vi "RC_Client Client 2.vi"(8 "error in (no error)":errorcluster) -> (0 "error out":errorcluster)   [LabVIEW 2019, in "RemoteControl.lvlib" / "RemoteControl.lvclass"]
uses:
  RemoteControl.lvclass
  a9d26567-5b45-42ca-bcd0-d9a82bf46199.vi
panel:
  in  "RemoteControl in":refnum<class "RemoteControl.lvclass">
  in  "milliseconds to wait":u32
  out "time (1 message) (ms)":u32
  out "messsages/s":dbl
  in  "remote port":u16=6341
  in  "address":string
  out "Parse Response":string
  out "Messages":i32
  in  "Stop":bool
  out "Command reponse":string
  out "Command":string
  out "commands":string[](array[string])
  # "CLIENT (API)"
  # "Connection info"
  # "Message Sent"
  # "Message Received"
  # "Metrics"
  # "client 2"
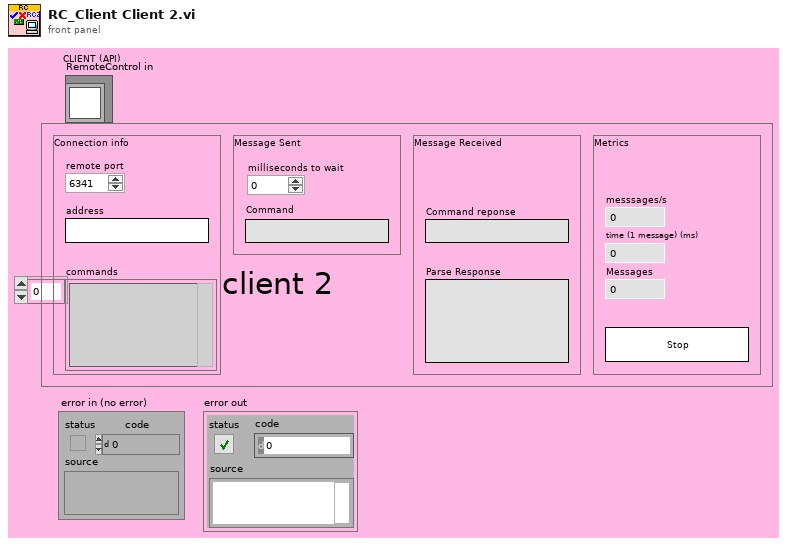
[diagram p1: front panel]
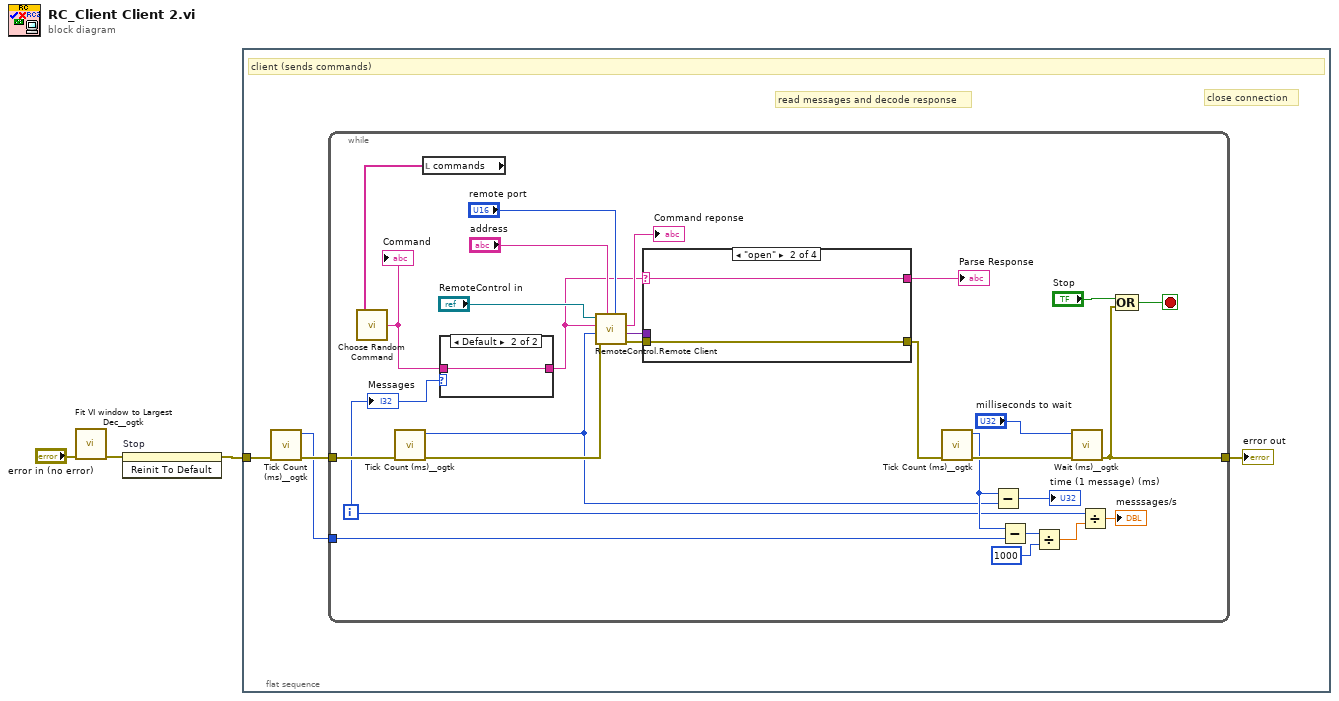
[diagram p0: block diagram]
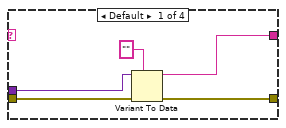
[diagram p2: hidden frame]
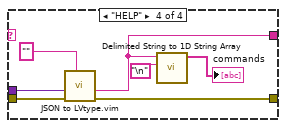
[diagram p4: hidden frame]
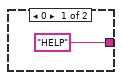
[diagram p5: hidden frame]
diagram:
  n1 = call <userlib>:"Fit VI window to Largest Dec__ogtk.vi"("error in (no error)"="error in (no error)") -> ("error out"=w3:errorcluster)  [unwired: 5 in, 1 out]
  n2 = invoke on="Stop" class="Bool" method="Reinit To Default"(error in=w3) -> (error out=w2:errorcluster)  [unwired: 2 in, 2 out]
  n3 = flat-sequence {
    tunnel: w2 -> [w4]
    frame #0 {
      # "close connection"
      # "read messages and decode response"
      # "client (sends commands)"
      n4 = call <userlib>:"Tick Count (ms)__ogtk.vi"("error in (no error)"=w4) -> ("error out"=w7:errorcluster, "millisecond timer value"=w6:u32)  [unwired: 9 in]
      n5 = while {
        tunnel: [w28] -> w5
        tunnel: w7 -> [w31]
        tunnel: w6 -> [w23]
        i -> [w20]
        stop <- w34 stop-if-true
        n6 = call <userlib>:"Tick Count (ms)__ogtk.vi"("error in (no error)"=w31) -> ("error out"=w21:errorcluster, "millisecond timer value"=w14:u32)  [unwired: 9 in]
        n7 = local read "commands"() -> (w16:string[])
        n8 = call "Choose Random Command.vi"("Array"=w16) -> ("String"=w15:string)
        "Command" <- w15
        n9 = case shown="Default" w20 {
          tunnel: ["HELP" ("Command") w52] -> w8
          tunnel: w15 -> [_ w52]
          frame 0 {
          }
          frame Default {
          }
        }
        n10 = call "RemoteControl.Remote Client.vi"("Port"="remote port", "address"="address", "error in (no error)"=w21, "Data"=w14, "Command"=w8, "RemoteControl in"="RemoteControl in") -> ("error out"=w11:errorcluster, "Data out"=w12:variant, "Command out"=→"Command reponse":string)  [unwired: 2 in, 1 out]
        n11 = case shown="\"open\"" w8 {
          selector: w8 -> [_ w40 w42 _]
          tunnel: [w35 w40 w42 w44] -> w10
          tunnel: w12 -> [w39 _ _ w48]
          tunnel: [w36 w41 w43 w45] -> w9
          tunnel: w11 -> [w37 w41 w43 w46]
          frame Default {
            n12 = Variant To Data(error in=w37, type="", Variant=w39) -> (data=w35:string, error out=w36:errorcluster)
          }
          frame "open" {
          }
          frame "close" {
          }
          frame "HELP" {
            n13 = call "JSON to LVtype.vim"("type"="", "error in (no error)"=w46, "JSON Data in"=w48) -> ("error out"=w45:errorcluster, "Data out"=w44:string)  [unwired: 7 in]
            n14 = call <vilib>:"Delimited String to 1D String Array.vi"("delimiter"="\n", "delimited string"=w44) -> ("string array"=→"commands":string[])  [unwired: 9 in]
          }
        }
        "Parse Response" <- w10
        n15 = call <userlib>:"Tick Count (ms)__ogtk.vi"("error in (no error)"=w9) -> ("error out"=w30:errorcluster, "millisecond timer value"=w25:u32)  [unwired: 9 in]
        n16 = Subtract(x=w25, y=w14) -> (x-y=→"time (1 message) (ms)":u32)
        n17 = Subtract(x=w25, y=w23) -> (x-y=w24:u32)
        n18 = Divide(x=w24, y=u32 1000) -> (x/y=w33:dbl)
        n19 = call <userlib>:"Wait (ms)__ogtk.vi"("error in (no error)"=w30, "milliseconds to wait"="milliseconds to wait") -> ("error out"=w28:errorcluster)  [unwired: 8 in, 1 out]
        n20 = Divide(x=w20, y=w33) -> (x/y=→"messsages/s":dbl)
        n21 = Compound Arithmetic op=OR("Stop", w28) -> (w34:bool)
        "Messages" <- w20
      }
      "error out" <- w5
    }
  }
